vi "Write Tags.vi"(8 "error in (no error)":errorcluster, 11 "State in":T1={"State"=enum."Idle", "Start Time"=timestamp(0 s since 1904-01-01), "Configuration"={"Cycle Period"=0.0, "Flow Meter Type"="", "Bronkhorst M13 Settings"={"VISA resource name"="", "Simulated?"=FALSE, "Smoothing Steps"=1}, "Bronkhorst M14 Settings"={"VISA resource name"="", "Simulated?"=FALSE, "Smoothing Steps"=1}}, "Current Time"=timestamp(0 s since 1904-01-01), "First Iteration"=FALSE, "Data"={"Flow Meter Read(g/min)"=0.0, "Density"=0.0, "Temp (C)"=0.0, "Totalized"=0.0}, "Process Name"="", "Log Started"=FALSE} {"Configuration"."Bronkhorst M14 Settings"."Smoothing Steps" min=1 step=1; "Configuration"."Bronkhorst M13 Settings"."Smoothing Steps" min=1 step=1}) -> (0 "error out":errorcluster, 3 "State out":T1={"State"=enum."Idle", "Start Time"=timestamp(0 s since 1904-01-01), "Configuration"={"Cycle Period"=0.0, "Flow Meter Type"="", "Bronkhorst M13 Settings"={"VISA resource name"="", "Simulated?"=FALSE, "Smoothing Steps"=1}, "Bronkhorst M14 Settings"={"VISA resource name"="", "Simulated?"=FALSE, "Smoothing Steps"=1}}, "Current Time"=timestamp(0 s since 1904-01-01), "First Iteration"=FALSE, "Data"={"Flow Meter Read(g/min)"=0.0, "Density"=0.0, "Temp (C)"=0.0, "Totalized"=0.0}, "Process Name"="", "Log Started"=FALSE} {"Configuration"."Bronkhorst M14 Settings"."Smoothing Steps" min=1 step=1; "Configuration"."Bronkhorst M13 Settings"."Smoothing Steps" min=1 step=1})   [LabVIEW 2018, in "Flow Module.lvlib" / "Flow Module Engine.lvlib"]
uses:
  Flow Module Engine.lvlib
  State Cluster.ctl
  State Enum.ctl
  Feed Module/Controls/Flow Module Settings Cluster.ctl
  Bronkhorst M13 Flow Meter/Settings Cluster.ctl
  Bronkhorst M14 Flow Meter/Settings Cluster.ctl
  Tag VIs/Tag FGV Operation Enum.ctl
  Shared Variables/Dynamic Shared Variables.lvlib
  Flow Module.lvlib
  Bronkhorst M13 Flow Meter/Bronkhorst M13 Flow Meter.lvlib
  Bronkhorst M14 Flow Meter/Bronkhorst M14 Flow Meter.lvlib
panel:
  # "Flow Meter Settings"
  # "Flow Meter Settings"
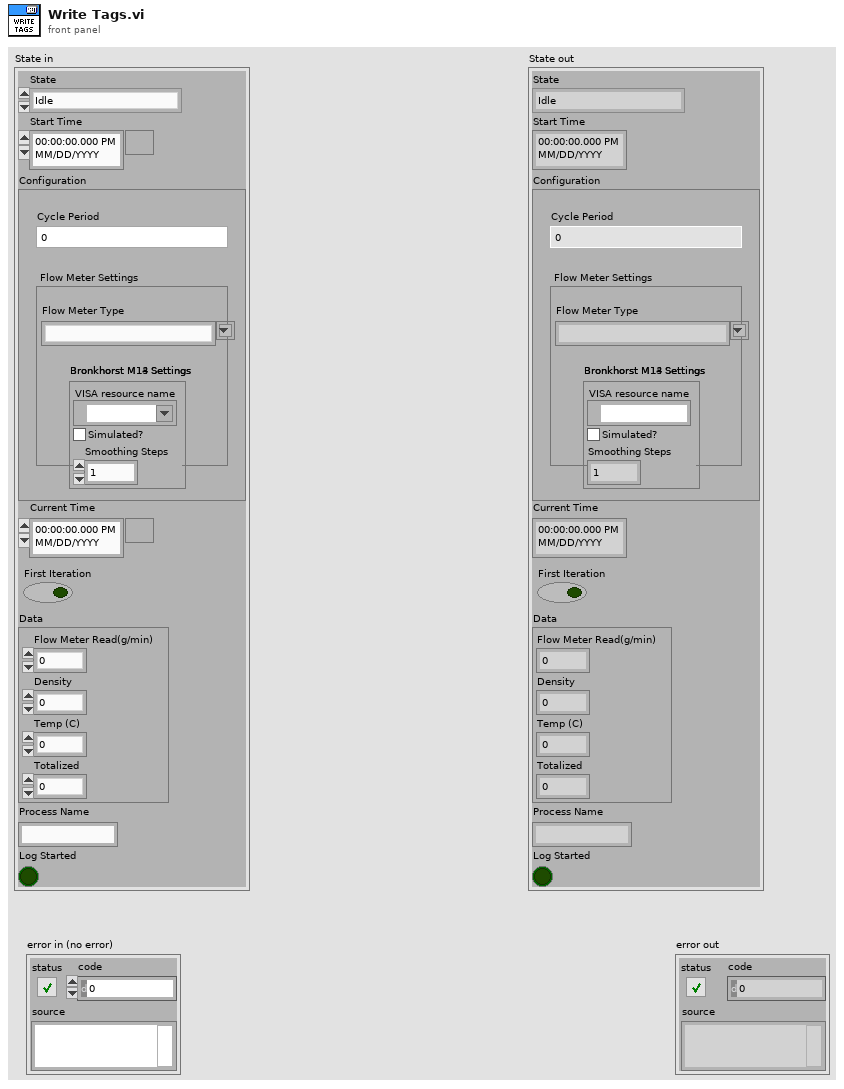
[diagram p1: front panel]
types:
  T1 = typedef "Flow Module.lvlib/Flow Module Engine.lvlib/State Cluster.ctl" = cluster{"State":T2, "Start Time":timestamp, "Configuration":T3, "Current Time":timestamp, "First Iteration":bool, "Data":cluster{"Flow Meter Read(g/min)":dbl, "Density":dbl, "Temp (C)":dbl, "Totalized":dbl}, "Process Name":string, "Log Started":bool}
  T2 = typedef "Flow Module.lvlib/Flow Module Engine.lvlib/State Enum.ctl" = enum16{"Measuring", "Idle"}
  T3 = typedef "Flow Module.lvlib/Flow Module Settings Cluster.ctl" = cluster{"Cycle Period":dbl, "Flow Meter Type":string, "Bronkhorst M13 Settings":T4, "Bronkhorst M14 Settings":T5}
  T4 = typedef "Bronkhorst M13 Flow Meter.lvlib/Settings Cluster.ctl" = cluster{"VISA resource name":refnum<visa-resource-name>, "Simulated?":bool, "Smoothing Steps":i32}
  T5 = typedef "Bronkhorst M14 Flow Meter.lvlib/Settings Cluster.ctl" = cluster{"VISA resource name":refnum<visa-resource-name>, "Simulated?":bool, "Smoothing Steps":i32}
  T6 = typedef "Tag FGV Operation Enum.ctl" = enum16{"Init", "Set Notification Queue", "Create Tag", "Commit", "Write Tag (Numeric)", "Write Tag (Boolean)", "Read All Tags", "Read One Tag", "Delete Tag Category", "Set Alarm Parameters (Numeric)", "Set Alarm Parameters (Boolean)", "Enable All Alarms", "Disable All Alarms", "Delete All Tags", "Read Alarms", "Ack Alarm", "Read Alarm Parameters (Numeric)", "Read Alarm Parameters (Boolean)"}
  T7 = typedef "Flow Module.lvlib/Tag Cluster.ctl" = cluster{"Flow Tag":string, "Density Tag":string, "Temp Tag":string, "Totalized Tag":string, "Input Disconnected":string, "Identifier Tag":string}
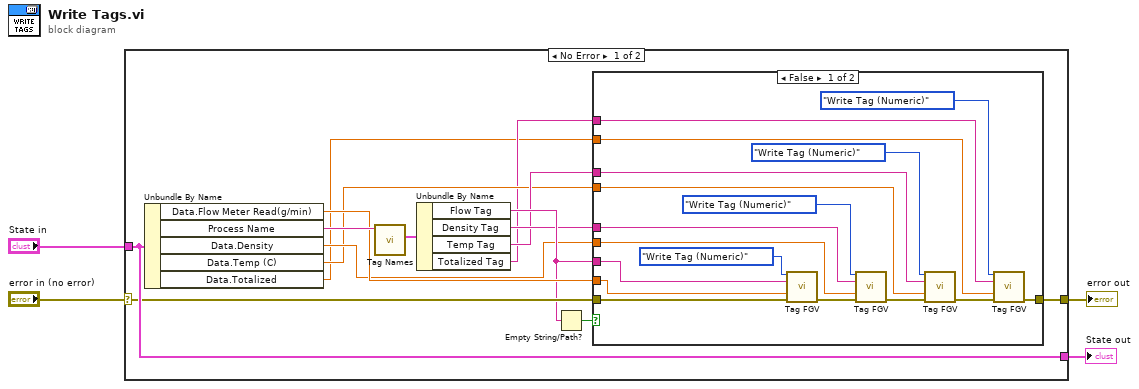
[diagram p0: block diagram]
diagram:
  n1 = case shown="No Error" "error in (no error)" {
    selector: "error in (no error)" -> [w14 w38]
    tunnel: [w17 w38] -> w3
    tunnel: "State in" -> [w15 w37]
    tunnel: [w15 w37] -> w1
    frame No Error {
      n2 = Unbundle By Name(w15) -> ("Data.Flow Meter Read(g/min)"=w13:dbl, "Process Name"=w18:string, "Data.Density"=w9:dbl, "Data.Temp (C)"=w7:dbl, "Data.Totalized"=w5:dbl)
      n3 = call "Tag Names.vi"("Process Name"=w18) -> ("Flow Tags"=w12:T7)  [unwired: 8 in, 2 out]
      n4 = Unbundle By Name(w12) -> ("Flow Tag"=w11:string, "Density Tag"=w10:string, "Temp Tag"=w8:string, "Totalized Tag"=w6:string)
      n5 = Empty String/Path?(string/path=w11) -> (empty?=w16:bool)
      n6 = case shown="False" w16 {
        tunnel: [w19 w36] -> w17
        tunnel: w14 -> [w34 w36]
        tunnel: w13 -> [w33 _]
        tunnel: w11 -> [w32 _]
        tunnel: w10 -> [w29 _]
        tunnel: w9 -> [w28 _]
        tunnel: w8 -> [w25 _]
        tunnel: w7 -> [w24 _]
        tunnel: w6 -> [w22 _]
        tunnel: w5 -> [w21 _]
        frame False {
          n7 = call "Tag FGV.vi"("Operation"=Tag_FGV_Operation_Enum."Write Tag (Numeric)", "Tag Name"=w32, "Data"=w33, "error in (no error)"=w34) -> ("error out"=w30:errorcluster)  [unwired: 4 in, 7 out]
          n8 = call "Tag FGV.vi"("Operation"=Tag_FGV_Operation_Enum."Write Tag (Numeric)", "Tag Name"=w29, "Data"=w28, "error in (no error)"=w30) -> ("error out"=w26:errorcluster)  [unwired: 4 in, 7 out]
          n9 = call "Tag FGV.vi"("Operation"=Tag_FGV_Operation_Enum."Write Tag (Numeric)", "Tag Name"=w25, "Data"=w24, "error in (no error)"=w26) -> ("error out"=w20:errorcluster)  [unwired: 4 in, 7 out]
          n10 = call "Tag FGV.vi"("Operation"=Tag_FGV_Operation_Enum."Write Tag (Numeric)", "Tag Name"=w22, "Data"=w21, "error in (no error)"=w20) -> ("error out"=w19:errorcluster)  [unwired: 4 in, 7 out]
        }
        frame True {
        }
      }
    }
    frame Error {
    }
  }
  "error out" <- w3
  "State out" <- w1
